vi "Send Toggle.vi"(8 "error in (no error)":errorcluster, 10 "Dirrection":enum16{"Forward", "Reverse"}(ring), 11 "Message queue":refnum<queue>) -> (0 "error out":errorcluster)   [LabVIEW 2015, in "Toggle.lvclass"]
uses:
  Toggle.lvclass
  Parent Message/Parent Message.lvclass
  Toggle.lvclass/Toggle.ctl
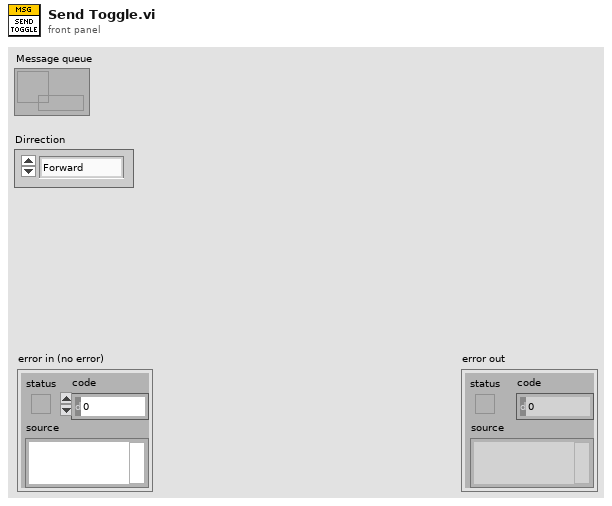
[diagram p1: front panel]
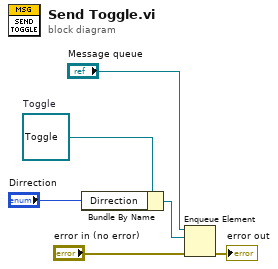
[diagram p0: block diagram]
diagram:
  w6 = refnum<class "Toggle.lvclass"> refnum  # Toggle
  n1 = Bundle By Name(cluster=w6, "Dirrection"="Dirrection") -> (w1:refnum<class "Toggle.lvclass">)
  n2 = Enqueue Element(queue="Message queue", element=w1, error in (no error)="error in (no error)") -> (error out=→"error out":errorcluster)  [unwired: 1 in, 2 out]
